vi "ExPairedMode.vi"() -> ()   [LabVIEW 2010]
panel:
  out "Paired Mode active":bool
  out "FF Avail":bool
  in  "Paired Mode":bool
  in  "Timing Mode":u32(ring)=1 items=["N/A", "Internal (Free Run)", "Trigger first (PM only)", "Ext Trig per exposure (Ext Sync)", "Ext Trig controls Exposure (PM only Bulb mode)", "Variable Ext Trigger Mode (PM only)", "Flash Mode (some PM only)"]
  in  "Exposure (sec)":dbl min=0.0 step=1e-06 format="%.6f"
  in  "stop":bool
  in  "Store":bool
  out "error out":errorcluster
  in  "error in (no error)":errorcluster
  # "ExPairedMode.vi\nThis example is for the CoolSnap HQ Dif camera\nIt shows the paired mode (DIF) operations in \ntwo windows at the same time."
  # "Indicators"
  # "Run Time Controls"
  # "Note1: Image is binned by 2"
  # "Note 2: Accum mode can't be run \nat the same time as paired mode"
  # "Note 3: 2nd display will appear on\ntop of first, you have to manually \nmove it over."
  # "Note 4:Trigger first works differently with paired \nmode, it does trigger per pair."
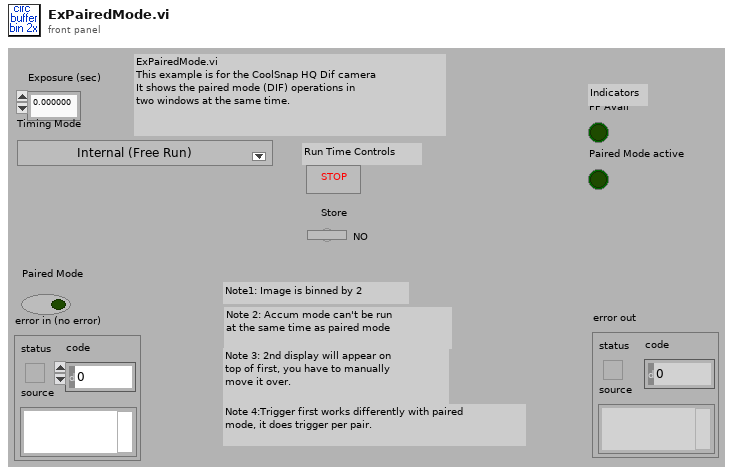
[diagram p1: front panel]
types:
  T1 = cluster{"acquire nframe mode":u32, "Exposure (sec)":dbl, "Number of Images":u32, "Software accumulation":u32}
  T2 = cluster{"Camera Handle":u32, "Pulser Handle":u32, "File Handle":u32, "Display Handle":u32, "Image Handle":u32}
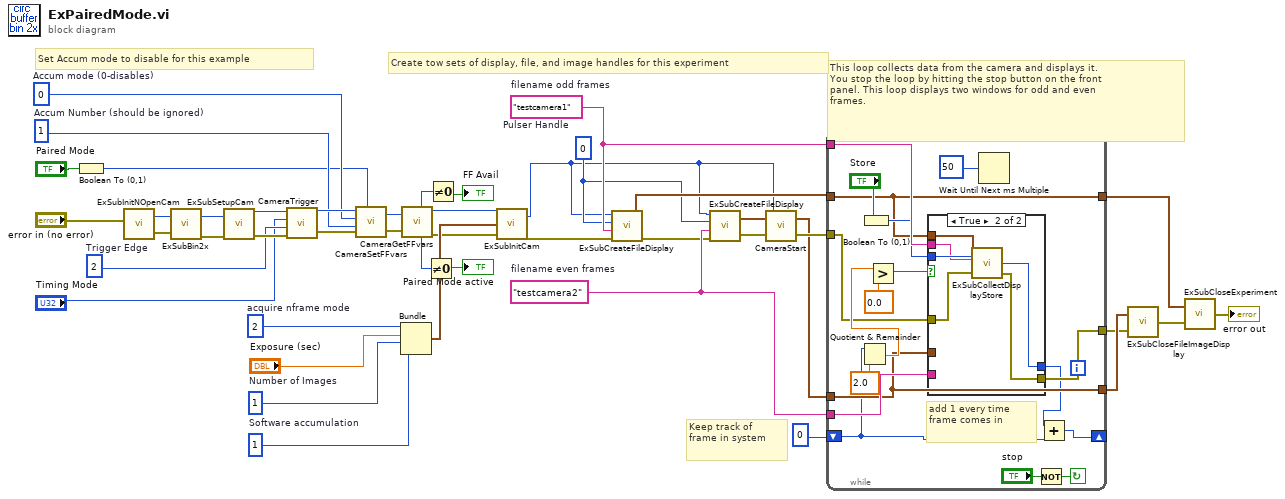
[diagram p0: block diagram]
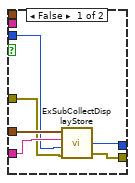
[diagram p2: hidden frame]
diagram:
  w15 = 1  # Accum Number (should be ignored)
  w16 = 0  # Accum mode (0-disables)
  w19 = "testcamera2"  # filename even frames
  w6 = u32 0  # Pulser Handle
  w31 = u32 2  # Trigger Edge
  w34 = u32 2  # acquire nframe mode
  w33 = u32 1  # Number of Images
  w32 = u32 1  # Software accumulation
  w44 = "testcamera1"  # filename odd frames
  # "This loop collects data from the camera and displays it.\nYou stop the loop by hitting the stop button on the front\npanel. This loop displays two windows for odd and even\nframes."
  # "Keep track of\nframe in system"
  # "Create tow sets of display, file, and image handles for this experiment"
  # "Set Accum mode to disable for this example"
  n1 = Boolean To (0,1)(Boolean="Paired Mode") -> (0, 1=w12:i16)
  n2 = call "ExSubInitNOpenCam.vi"("error in (no error)"="error in (no error)") -> ("Camera Handle"=w36:u32, "error out"=w35:errorcluster)
  n3 = call "ExSubBin2x.vi"("error in (no error)"=w35, "Camera Handle"=w36) -> ("error out"=w30:errorcluster, "Camera Handle"=w29:u32)
  n4 = call "ExSubSetupCam.vi"("error in (no error)"=w30, "Camera Handle"=w29) -> ("error out"=w38:errorcluster, "Camera Handle"=w39:u32)
  n5 = call <userlib>:"CameraTrigger.vi"("error in"=w38, "Trigger Edge"=w31, "Timing Mode"="Timing Mode", "Camera Handle"=w39) -> ("error out"=w24:errorcluster, "Camera Handle"=w23:u32)
  n6 = call <userlib>:"CameraSetFFvars.vi"(0:w23, 1:w16, 2:w15, 3:w24, 4:w12) -> (5:w26:u32, 6:w25:errorcluster)
  n7 = Bundle("acquire nframe mode"=w34, "Exposure (sec)"="Exposure (sec)", "Number of Images"=w33, "Software accumulation"=w32) -> (w41:T1)  [unwired: 1 in]
  n8 = call <userlib>:"CameraGetFFvars.vi"(0:w26, 1:w25) -> (2:w11:u8, 3:w9:u32, 4:w28:u32, 7:w27:errorcluster)  [unwired: 2 out]
  n9 = Not Equal To 0?(x=w9) -> (x != 0?=→"Paired Mode active":bool)
  n10 = Not Equal To 0?(x=w11) -> (x != 0?=→"FF Avail":bool)
  n11 = call "ExSubInitCam.vi"("error in (no error)"=w27, "Camera Information"=w41, "Camera Handle"=w28) -> ("error out"=w22:errorcluster, "Camera Handle"=w5:u32)
  n12 = call "ExSubCreateFileDisplay.vi"("error in (no error)"=w22, "File and Display Name"=w44, "Pulser Handle"=w6, "Camera Handle"=w5) -> ("error out"=w7:errorcluster, "Handles Out"=w40:T2)
  n13 = call "ExSubCreateFileDisplay.vi"("error in (no error)"=w7, "File and Display Name"=w19, "Pulser Handle"=w6, "Camera Handle"=w5) -> ("error out"=w21:errorcluster, "Handles Out"=w20:T2)
  n14 = call <userlib>:"CameraStart.vi"("error in"=w21, "Camera Handle"=w5) -> ("error out"=w37:errorcluster)  [unwired: 1 out]
  n15 = while {
    tunnel: w40 -> [w49]
    tunnel: w37 -> [w52]
    tunnel: w44 -> [w57]
    tunnel: [w50] -> w1
    tunnel: [w49] -> w3
    tunnel: w20 -> [w48]
    tunnel: w19 -> [w51]
    tunnel: [w48] -> w4
    shift-right: [w47] -> _
    shift-left: 0 -> [w45]
    stop <- w60 continue-if-true
    # "add 1 every time\nframe comes in"
    n16 = Quotient & Remainder(x=w45, y=2.0) -> (x-y*floor(x/y)=w54:dbl)  [unwired: 1 out]
    n17 = Boolean To (0,1)(Boolean="Store") -> (0, 1=w56:i16)
    n18 = Greater?(x=w54, y=0.0) -> (0:w55:bool)
    n19 = case shown="True" w55 {
      tunnel: w57 -> [_ w72]
      tunnel: w49 -> [_ w73]
      tunnel: w56 -> [w66 w74]
      tunnel: w52 -> [w65 w71]
      tunnel: w48 -> [w68 _]
      tunnel: w51 -> [w67 _]
      tunnel: [w64 w70] -> w50
      tunnel: [w63 w69] -> w46
      frame False {
        n20 = call "ExSubCollectDisplayStore.vi"("error in (no error)"=w65, "Store flag"=w66, "Display Title"=w67, "Handle Cluster"=w68) -> ("error out"=w64:errorcluster, "got frame"=w63:u32)  [unwired: 1 out]
      }
      frame True {
        n21 = call "ExSubCollectDisplayStore.vi"("error in (no error)"=w71, "Store flag"=w74, "Display Title"=w72, "Handle Cluster"=w73) -> ("error out"=w70:errorcluster, "got frame"=w69:u32)  [unwired: 1 out]
      }
    }
    n22 = Wait Until Next ms Multiple(millisecond multiple=u32 50) -> ()  [unwired: 1 out]
    n23 = Not(x="stop") -> (.not. x?=w60:bool)
    n24 = Add(x=w46, y=w45) -> (x+y=w47:u32)
  }
  n25 = call "ExSubCloseFileImageDisplay.vi"("error in (no error)"=w1, "Handles In"=w4) -> ("error out"=w2:errorcluster)
  n26 = call "ExSubCloseExperiment.vi"("error in (no error)"=w2, "Handles In"=w3) -> ("error out"=→"error out":errorcluster)
